vi "Get All Route points.vi"(7 "Altitude (m)":sgl=10.0, 8 "Error In":errorcluster, 11 "Route Index":i32) -> (0 "Error Out":errorcluster, 3 "Waypoints":T1[](array[typedef]))   [LabVIEW 2014]
uses:
  MAVLink/Controls/Mission Planning Controls/MAVLINK Mission Item.ctl
  MAVLink/Controls/MAVLINK Mav Frame.ctl
  C:/Robotic Systems/Products/Surveyor/Software/Ground Station/Data/Mapping DLL/GMap.NET.WindowsForms.dll
  Data/Mapping DLL/GMap.NET.WindowsForms.dll
  C:/Robotic Systems/Products/Surveyor/Software/Ground Station/Data/Mapping DLL/GMap.NET.Core.dll
  Data/Mapping DLL/GMap.NET.Core.dll
  Reference/SubVI/GMap DLL Refernce.vi
  Reference/SubVI/Main Map Control Refernce.vi
  Aircraft Information/Sub VI/Selected Aircraft/SubVI/Get Selected Aircraft.vi
  Aircraft Information/Sub VI/Get Aircraft GPS.vi
  MAVLink/Commands/Mission Planning/MISSION_ITEM SubVI/MISSION_ITEM Land.vi
  MAVLink/Commands/Mission Planning/MISSION_ITEM SubVI/MISSION_ITEM Loiter (Time).vi
  MAVLink/Commands/Mission Planning/MISSION_ITEM SubVI/MISSION_ITEM Takeoff.vi
  MAVLink/Commands/Mission Planning/MISSION_ITEM SubVI/MISSION_ITEM Waypoint.vi
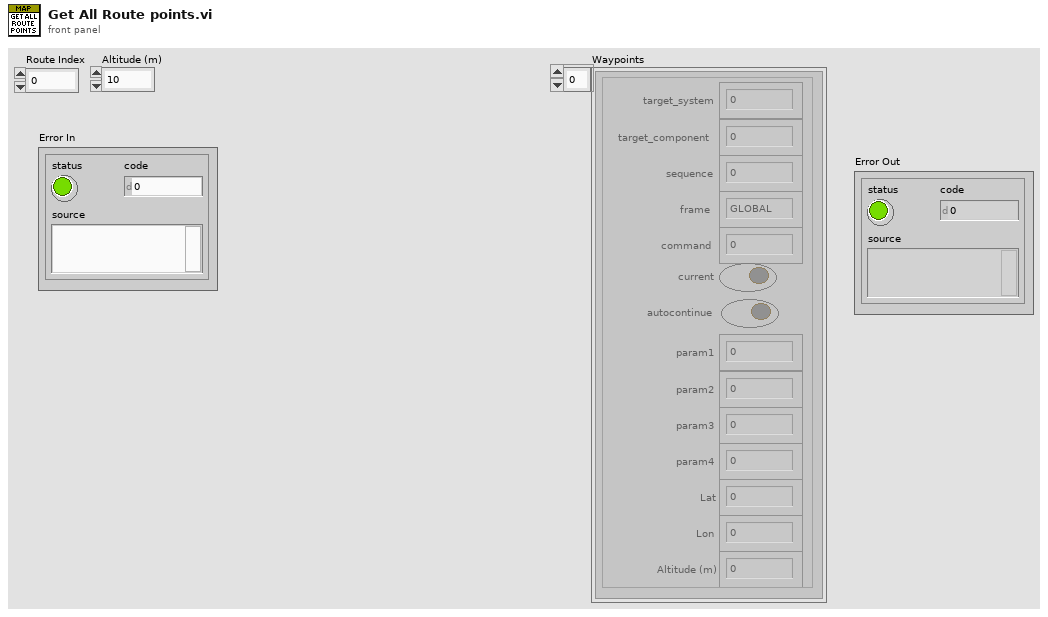
[diagram p1: front panel]
types:
  T1 = typedef "MAVLINK Mission Item.ctl" = cluster{"target_system":u8, "target_component":u8, "sequence":u16, "frame":T2, "command":u16, "current":bool, "autocontinue":bool, "param1":sgl, "param2":sgl, "param3":sgl, "param4":sgl, "Lat":sgl, "Lon":sgl, "Altitude (m)":sgl}
  T2 = typedef "MAVLINK Mav Frame.ctl" = enum8{"GLOBAL", "LOCAL NED", "MISSION", "GLOBAL RELATIVE ALT", "LOCAL ENU", "GLOBAL INT", "GLOBAL RELATIVE ALT INT", "LOCAL OFFSET NED", "BODY NED", "BODY OFFSET NED", "GLOBAL TERRAIN ALT", "GLOBAL TERRAIN ALT INT"}
  T3 = typedef "Aircraft GPS Data.ctl" = cluster{"Latitude (degrees)":dbl, "Longitude (degrees)":dbl, "Altitude (m)":dbl, "Fix Type":u8, "HDOP (cm)":u16, "VDOP (cm)":u16, "Ground Speed (m/s)":dbl, "Coarse Over Ground (degrees)":u16, "Number of Satellites":u8}
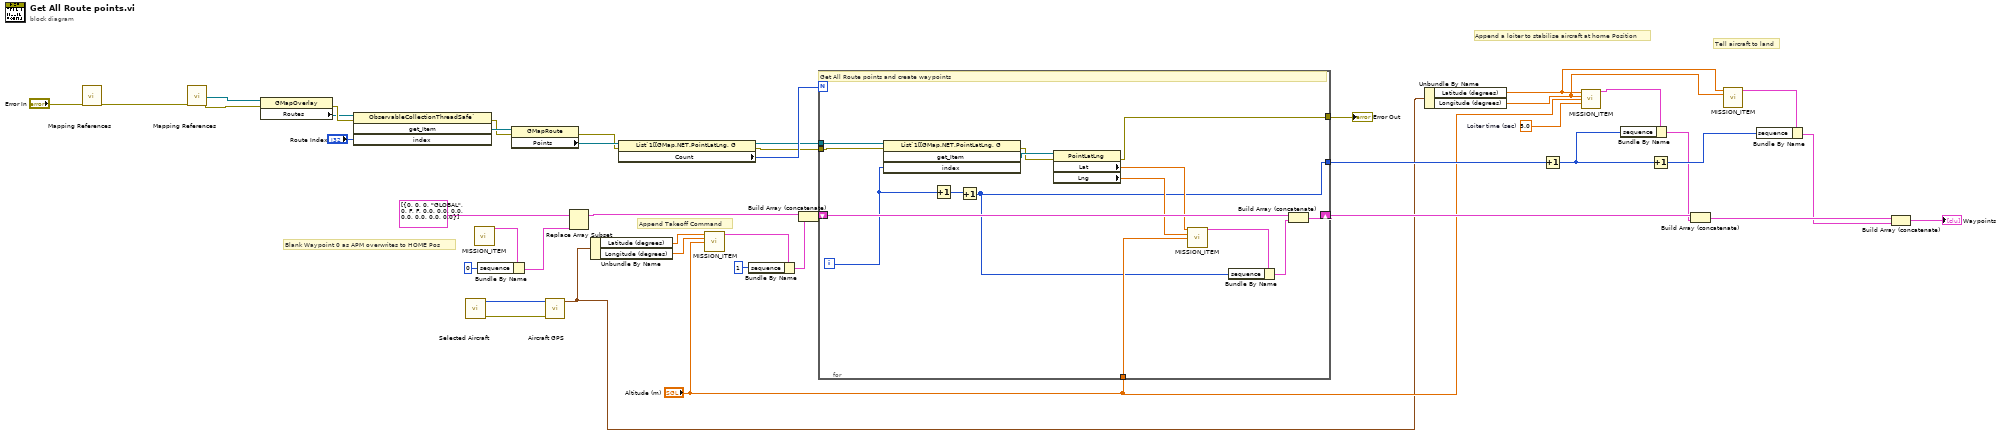
[diagram p0: block diagram]
diagram:
  w13 = sgl 5.0  # Loiter time (sec)
  # "Blank Waypoint 0 as APM overwrites to HOME Pos"
  # "Append Takeoff Command"
  # "Tell aircraft to land"
  # "Append a loiter to stabilise aircraft at home Position"
  n1 = call-poly "Mapping References.vi"("Error In"="Error In") -> ("Error Out"=w37:errorcluster)  [unwired: 9 in, 1 out]
  n2 = call-poly "Mapping References.vi"("Error In"=w37) -> ("Error Out"=w39:errorcluster, "Main Map Reference"=w38:refnum<k24>)  [unwired: 9 in]
  n3 = property class="GMapOverlay"(reference=w38, error in=w39) -> (error out=w43:errorcluster, "Routes"=w40:refnum<k24>)  [unwired: 1 out]
  n4 = invoke class="ObservableCollectionThreadSafe`" method="get_Item"(reference=w40, error in=w43, "index"="Route Index") -> (error out=w35:errorcluster, "get_Item"=w41:refnum<k24>)  [unwired: 1 in, 2 out]
  n5 = call-poly "Selected Aircraft.vi"() -> ("Error Out"=w19:errorcluster, "Selected Aircraft ID Out"=w18:u8)  [unwired: 10 in]
  n6 = call-poly "MISSION_ITEM.vi"() -> ("Mission Item"=w3:T1)  [unwired: 15 in]
  n7 = Bundle By Name(cluster=w3, "sequence"=u16 0) -> (w1:T1)
  n8 = property class="GMapRoute"(reference=w41, error in=w35) -> (error out=w33:errorcluster, "Points"=w34:refnum<k24>)  [unwired: 1 out]
  n9 = call-poly "Aircraft GPS.vi"("Error In"=w19, "Aircraft ID"=w18) -> ("Aircraft Att Data Out"=w5:T3)  [unwired: 8 in, 1 out]
  n10 = Replace Array Subset(array=T1[] [{"target_system"=0, "target_component"=0, "sequence"=0, "frame"=enum."GLOBAL", "command"=0, "current"=FALSE, "autocontinue"=FALSE, "param1"=0.0, "param2"=0.0, "param3"=0.0, "param4"=0.0, "Lat"=0.0, "Lon"=0.0, "Altitude (m)"=0.0}], new element=w1) -> (w20:T1[])  [unwired: 1 in]
  n11 = Unbundle By Name(w5) -> ("Latitude (degrees)"=w16:dbl, "Longitude (degrees)"=w15:dbl)
  n12 = property class="List`1[[GMap.NET.PointLatLng, G"(reference=w34, error in=w33) -> (reference out=w31:refnum<k24>, error out=w22:errorcluster, "Count"=w32:i32)
  n13 = call-poly "MISSION_ITEM.vi"("Lat"=w16, "Lon"=w15, "Altitude (m)"="Altitude (m)") -> ("Mission Item"=w17:T1)  [unwired: 12 in]
  n14 = Bundle By Name(cluster=w17, "sequence"=u16 1) -> (w23:T1)
  n15 = Build Array (concatenate)(w20, w23) -> (w24:T1[])
  n16 = for {
    N: w32 -> [_]
    tunnel: w31 -> [w58]
    shift-right: [w56] -> w29
    shift-left: w24 -> [w57]
    tunnel: [w53] -> w4
    tunnel: [w44] -> w30
    tunnel: "Altitude (m)" -> [w47]
    tunnel: w22 -> [w50]
    i -> [w52]
    # "Get All Route points and create waypoints"
    n17 = invoke class="List`1[[GMap.NET.PointLatLng, G" method="get_Item"(reference=w58, error in=w50, "index"=w52) -> (error out=w54:errorcluster, "get_Item"=w55:refnum<k24>)  [unwired: 1 in, 2 out]
    n18 = Increment(x=w52) -> (x+1=w51:i32)
    n19 = Increment(x=w51) -> (x+1=w44:i32)
    n20 = property class="PointLatLng"(reference=w55, error in=w54) -> (error out=w53:errorcluster, "Lat"=w49:dbl, "Lng"=w48:dbl)  [unwired: 1 out]
    n21 = call-poly "MISSION_ITEM.vi"("Lat"=w49, "Lon"=w48, "Altitude (m)"=w47) -> ("Mission Item"=w46:T1)  [unwired: 12 in]
    n22 = Bundle By Name(cluster=w46, "sequence"=w44) -> (w45:T1)
    n23 = Build Array (concatenate)(w57, w45) -> (w56:T1[])
  }
  "Error Out" <- w4
  n24 = Unbundle By Name(w5) -> ("Latitude (degrees)"=w8:dbl, "Longitude (degrees)"=w7:dbl)
  n25 = Increment(x=w30) -> (x+1=w11:i32)
  n26 = call-poly "MISSION_ITEM.vi"("Lat"=w8, "Lon"=w7, "Altitude (m)"="Altitude (m)", "Loiter time (sec)"=w13) -> ("Mission Item"=w12:T1)  [unwired: 11 in]
  n27 = Bundle By Name(cluster=w12, "sequence"=w11) -> (w10:T1)
  n28 = Increment(x=w11) -> (x+1=w25:i32)
  n29 = Build Array (concatenate)(w29, w10) -> (w27:T1[])
  n30 = call-poly "MISSION_ITEM.vi"("Lat"=w8, "Lon"=w7) -> ("Mission Item"=w9:T1)  [unwired: 13 in]
  n31 = Bundle By Name(cluster=w9, "sequence"=w25) -> (w26:T1)
  n32 = Build Array (concatenate)(w27, w26) -> (→"Waypoints":T1[])
